vi "CheckCollision.vi"(8 "error in":errorcluster, 10 "sprite in":refnum<class "Sprite.lvclass">, 11 "class data in":refnum<class "SceneObject.lvclass">) -> (0 "error out":errorcluster, 1 "collisionInfo out":cluster{"collision":bool, "fatal":bool}, 2 "sprite out":refnum<class "Sprite.lvclass">, 3 "class data out":refnum<class "SceneObject.lvclass">)   [LabVIEW 2010, in "RenderBase.lvlib" / "SceneObject.lvclass"]
doc: "Checks for a collision. This is not an abstract method but a default implementation that does nothing (not every scene object might need a collision check). It must be overridden by a child class to implement a particular collision check."
uses:
  SceneObject.lvclass
  Sprite_class/Sprite.lvclass
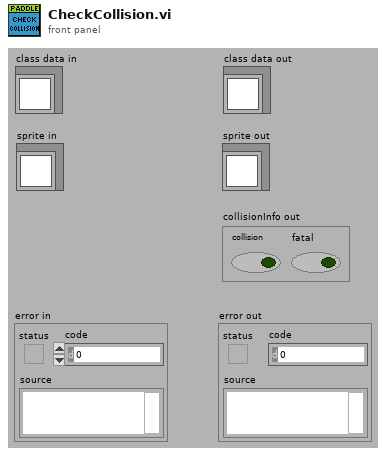
[diagram p1: front panel]
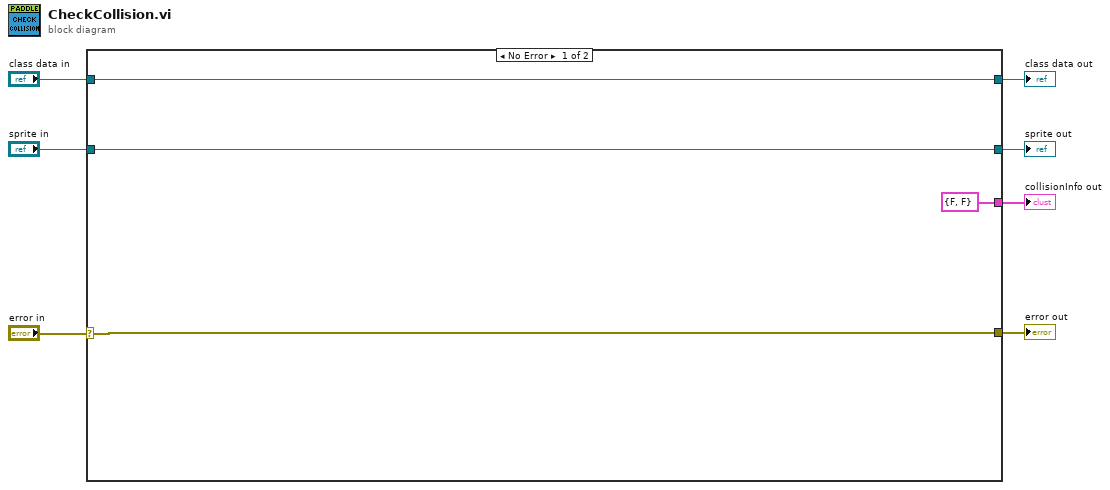
[diagram p0: block diagram]
diagram:
  n1 = case shown="No Error" "error in" {
    selector: "error in" -> [w8 w14]
    tunnel: [w8 w14] -> w7
    tunnel: "sprite in" -> [w10 w12]
    tunnel: [w11 w13] -> w5
    tunnel: "class data in" -> [w11 w13]
    tunnel: [w10 w12] -> w2
    tunnel: [cluster{"collision":bool, "fatal":bool} {"collision"=FALSE, "fatal"=FALSE} ("collisionInfo out") _] -> w1
    frame No Error {
    }
    frame Error {
    }
  }
  "error out" <- w7
  "class data out" <- w5
  "sprite out" <- w2
  "collisionInfo out" <- w1
